vi "LeidosBarCode_DataBaseParser.vi"(0 "BarCode_In":string, 7 "Rev_suffix":string) -> (1 "Desc":string, 2 "BC_ESN":string="0x00003609B620", 3 "BarCode_Out":string, 4 "Company":string="RaGE Systems", 6 "BC_MSN":string="TA22240078", 8 "Rage PN":string="5083561", 10 "LotID":string="2224", 12 "rev_c?(t)":bool, 13 "BarCodeInfo":string="#RaGE Systems\r\n#Prod_Name: Wideband Antenna Module\r\n#Rage_PN: 5083561\r\n#Revision: C.01\r\n#LotID: 2224\r\n#MSN: TA22240078\r\n#ESN: 0x00003609B620\r\n", 14 "Revision":string="C.01", 15 "Success?(t)":bool)   [LabVIEW 2018]
uses:
  Initialize References/Sequence Globals.vi
panel:
  out "py script path":string
  out "vi name(str)":string
  out "standard output":string
  out "error out":errorcluster
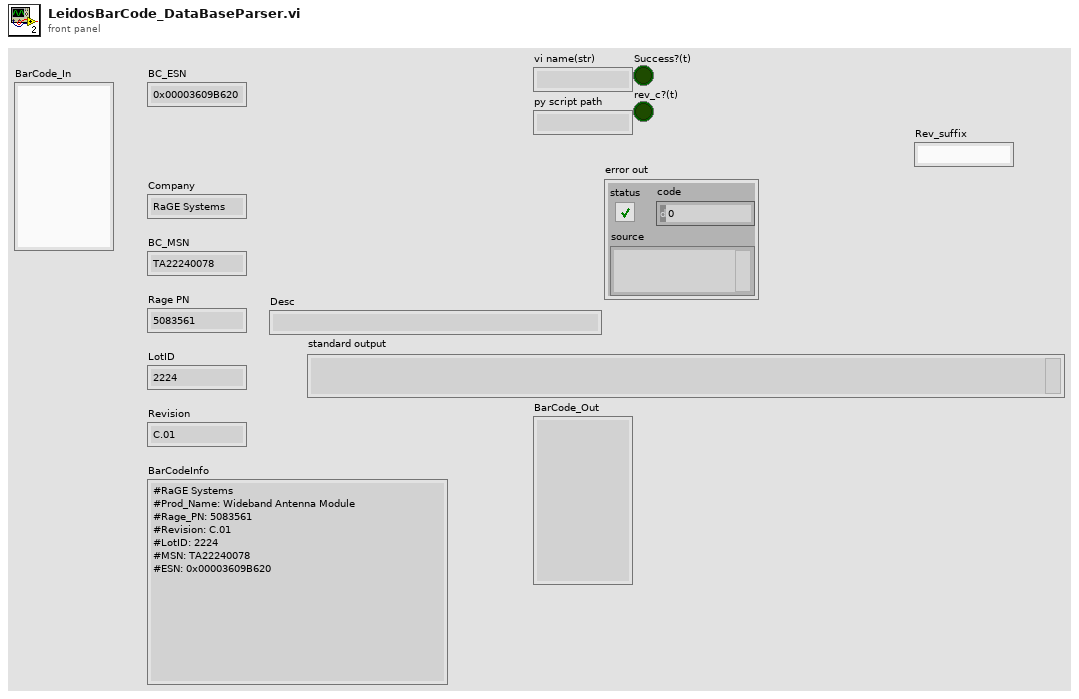
[diagram p1: front panel]
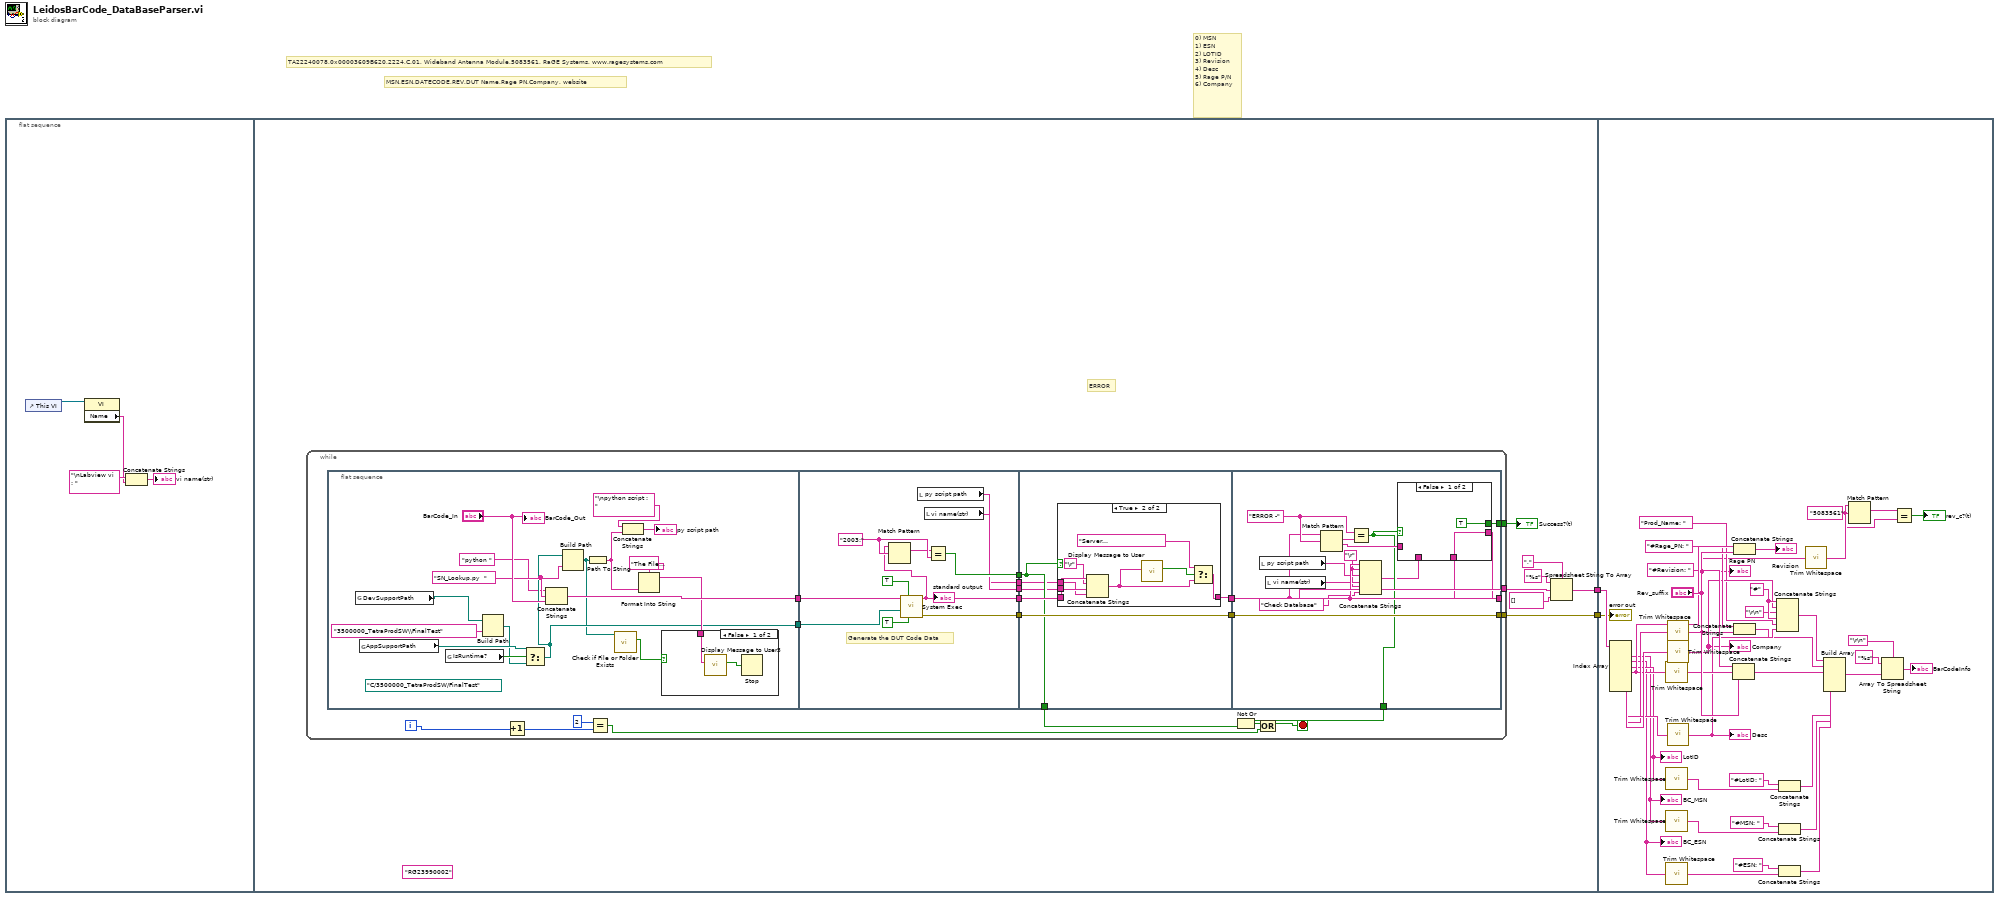
[diagram p0: block diagram]
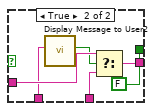
[diagram p4: hidden frame]
diagram:
  # "0) MSN\n1) ESN\n2) LOTID\n3) Revision \n4) Desc\n5) Rage P/N\n6) Company"
  # "MSN,ESN,DATECODE,REV,DUT Name,Rage PN,Company, website"
  # "TA22240078,0x00003609B620,2224,C.01, Wideband Antenna Module,5083561, RaGE Systems, www.ragesystems.com"
  n1 = flat-sequence {
    tunnel: [w10] -> w2
    tunnel: [w9] -> w1
    tunnel: w2 -> [w127]
    tunnel: w1 -> [w105]
    frame #0 {
      n2 = control-ref of="This VI"() -> (w6:refnum<vi>)
      n3 = property class="VI"(reference=w6) -> ("Name"=w4:string)  [unwired: 1 in, 2 out]
      n4 = Concatenate Strings("\nLabview vi : " ("string"), w4) -> (→"vi name(str)":string)
    }
    frame #1 {
      (unwired) "RG23990002" ("LD_BarCode_In")
      # "ERROR"
      n5 = while {
        tunnel: [w26] -> w9
        tunnel: [w25] -> w8
        tunnel: [w14] -> w7
        i -> [w20]
        stop <- w21 stop-if-true
        n6 = flat-sequence {
          tunnel: [w50] -> w33
          tunnel: [w39] -> w32
          tunnel: w33 -> [w63]
          tunnel: w32 -> [w62]
          tunnel: [w59] -> w31
          tunnel: [w56] -> w30
          tunnel: [w55] -> w29
          tunnel: [w54] -> w16
          tunnel: [w53] -> w15
          tunnel: w31 -> [w69]
          tunnel: w30 -> [w68]
          tunnel: w29 -> [w66]
          tunnel: [w69] -> w28
          tunnel: [w67] -> w27
          tunnel: [w66] -> w22
          tunnel: w16 -> [w65]
          tunnel: w15 -> [w64]
          tunnel: [w88] -> w25
          tunnel: [w91] -> w26
          tunnel: w28 -> [w91]
          tunnel: w27 -> [w85]
          tunnel: [w86] -> w23
          tunnel: [w79] -> w14
          frame #0 {
            w48 = "SN_Lookup.py  " ("command line")
            (unwired) path "C:/3500000_TetraProdSW/FinalTest" ("working directory")
            n7 = global read "Sequence Globals.vi" "DevSupportPath"() -> (w36:path)
            n8 = global read "Sequence Globals.vi" "AppSupportPath"() -> (w44:path)
            n9 = global read "Sequence Globals.vi" "IsRuntime?"() -> (w45:bool)
            n10 = Build Path(base path=w36, name or relative path="3500000_TetraProdSW\\FinalTest") -> (appended path=w37:path)
            n11 = Select(t=w44, s=w45, f=w37) -> (s? t:f=w39:path)
            n12 = Concatenate Strings("python " ("command line"), w48, "BarCode_In") -> (w50:string)
            n13 = Build Path(base path=w39, name or relative path=w48) -> (appended path=w34:path)
            n14 = Path To String(path=w34) -> (string=w41:string)
            n15 = call <vilib>:"Check if File or Folder Exists.vi"("path"=w34) -> ("file or folder exists?"=w43:bool)  [unwired: 8 in, 2 out]
            n16 = Concatenate Strings("\npython script : " ("string"), w41) -> (→"py script path":string)
            n17 = Format Into String(format string="The File : %s cant be found.\nCancelling", w41) -> (resulting string=w40:string)  [unwired: 2 in, 1 out]
            n18 = case shown="False" w43 {
              tunnel: w40 -> [w51 _]
              frame False {
                n19 = call "Display Message to User3"("Message"=w51) -> ("STOP"=w52:bool)  [unwired: 9 in, 1 out]
                n20 = Stop(stop? (T)=w52) -> ()
              }
              frame True {
              }
            }
            "BarCode_Out" <- "BarCode_In"
          }
          frame #1 {
            w61 = "2003:" ("regular expression")
            # "Generate the DUT Code Data"
            n21 = call <vilib>:"System Exec.vi"("run minimized? (F)"=TRUE, "wait until completion? (T)"=TRUE, "working directory"=w62, "command line"=w63) -> ("error out"=w59:errorcluster, "standard output"=w56:string)  [unwired: 4 in, 2 out]
            "standard output" <- w56
            n22 = Match Pattern(string=w56, regular expression=w61) -> (match substring=w60:string)  [unwired: 1 in, 3 out]
            n23 = local read "py script path"() -> (w54:string)
            n24 = local read "vi name(str)"() -> (w53:string)
            n25 = Equal?(x=w60, y=w61) -> (x = y?=w55:bool)
          }
          frame #2 {
            n26 = case shown="True" w66 {
              tunnel: w68 -> [w70 w77]
              tunnel: [w70 w76] -> w67
              tunnel: w65 -> [_ w72]
              tunnel: w64 -> [_ w71]
              frame False {
              }
              frame True {
                n27 = Concatenate Strings(w77, "\r", w72, w71) -> (w74:string)
                n28 = call "Display Message to User"("Message"=w74) -> ("OK"=w75:bool)  [unwired: 9 in, 1 out]
                n29 = Select(t="Server Error,Error,Error,Error,Error,Error,Error, Error", s=w75, f=w74) -> (s? t:f=w76:string)
              }
            }
          }
          frame #3 {
            w81 = "\r"
            w89 = "ERROR -" ("regular expression")
            n30 = local read "py script path"() -> (w84:string)
            n31 = local read "vi name(str)"() -> (w83:string)
            n32 = Match Pattern(string=w85, regular expression=w89) -> (match substring=w90:string, after substring=w87:string)  [unwired: 1 in, 2 out]
            n33 = Equal?(x=w89, y=w90) -> (x = y?=w86:bool)
            n34 = Concatenate Strings(w85, w81, w84, w83, w81, "Check Database" ("string")) -> (w82:string)
            n35 = case shown="False" w86 {
              tunnel: [w93 w99] -> w88
              tunnel: w85 -> [w93 w98]
              tunnel: w87 -> [_ w97]
              tunnel: w82 -> [_ w95]
              tunnel: [TRUE ("Success?(t)") FALSE ("Success?(t)")] -> w79
              frame False {
              }
              frame True {
                n36 = call "Display Message to User2"("Message"=w95) -> ("OK"=w96:bool)  [unwired: 9 in, 1 out]
                n37 = Select(t=w97, s=w96, f=w98) -> (s? t:f=w99:string)
              }
            }
          }
        }
        n38 = Increment(x=w20) -> (x+1=w19:i32)
        n39 = Equal?(x=2, y=w19) -> (x = y?=w17:bool)
        n40 = Not Or(1:w22, 2:w23) -> (0:w24:bool)
        n41 = Or(x=w24, y=w17) -> (x .or. y?=w21:bool)
      }
      "Success?(t)" <- w7
      n42 = Spreadsheet String To Array(delimiter (Tab)=",", format string="%s", spreadsheet string=w8, array type (2D Dbl)=string[] []) -> (array=w10:string[])
    }
    frame #2 {
      w101 = "5083561" ("regular expression")
      w121 = "#" ("string")
      n43 = Index Array(array=w127) -> (element #1=w131:string, element #2=w132:string, element #3=w133:string, element #4=w134:string, element #5=w136:string, element #6=w135:string, element #7=w137:string)  [unwired: 7 in]
      "BC_MSN" <- w131
      "LotID" <- w133
      "BC_ESN" <- w132
      n44 = call <vilib>:"Trim Whitespace.vi"("string"=w134) -> ("trimmed string"=w130:string)  [unwired: 1 in]
      n45 = call <vilib>:"Trim Whitespace.vi"("string"=w133) -> ("trimmed string"=w129:string)  [unwired: 1 in]
      n46 = call <vilib>:"Trim Whitespace.vi"("string"=w131) -> ("trimmed string"=w128:string)  [unwired: 1 in]
      n47 = call <vilib>:"Trim Whitespace.vi"("string"=w132) -> ("trimmed string"=w111:string)  [unwired: 1 in]
      n48 = call <vilib>:"Trim Whitespace.vi"("string"=w135) -> ("trimmed string"=w104:string)  [unwired: 1 in]
      "Rage PN" <- w104
      n49 = call <vilib>:"Trim Whitespace.vi"("string"=w137) -> ("trimmed string"=w120:string)  [unwired: 1 in]
      "Company" <- w120
      n50 = call <vilib>:"Trim Whitespace.vi"("string"=w136) -> ("trimmed string"=w122:string)  [unwired: 1 in]
      "Desc" <- w122
      n51 = Concatenate Strings("#Revision: ", w130, "Rev_suffix") -> (w108:string)
      n52 = Concatenate Strings(w134, "Rev_suffix") -> (→"Revision":string)
      n53 = Concatenate Strings("#Rage_PN: ", w104) -> (w109:string)
      n54 = Concatenate Strings(w121, w120, "\r\n", w121, "Prod_Name: " ("string"), w122) -> (w110:string)
      n55 = Concatenate Strings("#LotID: ", w129) -> (w107:string)
      n56 = Concatenate Strings("#MSN: ", w128) -> (w106:string)
      n57 = Concatenate Strings("#ESN: ", w111) -> (w117:string)
      n58 = call <vilib>:"Trim Whitespace.vi"("string"=w104) -> ("trimmed string"=w103:string)  [unwired: 1 in]
      n59 = Build Array(w110, w109, w108, w107, w106, w117) -> (w115:string[])
      n60 = Match Pattern(string=w103, regular expression=w101) -> (match substring=w102:string)  [unwired: 1 in, 3 out]
      n61 = Array To Spreadsheet String(delimiter (Tab)="\r\n", array=w115, 3:"%s" ("format string")) -> (spreadsheet string=→"BarCodeInfo":string)
      n62 = Equal?(x=w102, y=w101) -> (x = y?=→"rev_c?(t)":bool)
      "error out" <- w105
    }
  }
